vi "DataBasePATH.vi"() -> (3 "DataBase path":path)   [LabVIEW 2020, in "DataBaseSQLlite.lvlib"]
uses:
  DataBaseSQLlite.lvlib
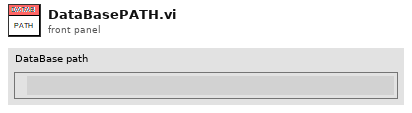
[diagram p1: front panel]
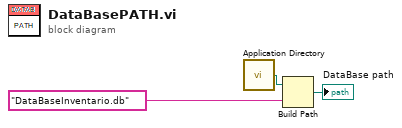
[diagram p0: block diagram]
diagram:
  n1 = call <vilib>:"Application Directory.vi"() -> ("Application Directory"=w3:path)
  n2 = Build Path(base path=w3, name or relative path="DataBaseInventario.db") -> (appended path=→"DataBase path":path)
